vi "TEST Set Wind Speeds - Solution.vi"() -> ()   [LabVIEW 2011]
doc: "Two VI solution that allows the user to test the Wind Turbine class. Speed is set in one VI and read in another.\n\nAAL 9/09"
uses:
  SEQ - Solution.lvlib
panel:
  in  "Exit":bool
  in  "Set Speed":bool
  in  "Turbine":u16(ring) items=["Wind Turbine #1", "Wind Turbine #2", "Wind Turbine #3"]
  in  "Wind Speed (m/s)":dbl
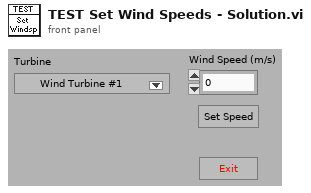
[diagram p1: front panel]
types:
  T1 = typedef "SEQ - Solution.lvlib/Wind Turbine DataRef.ctl" = refnum<queue>
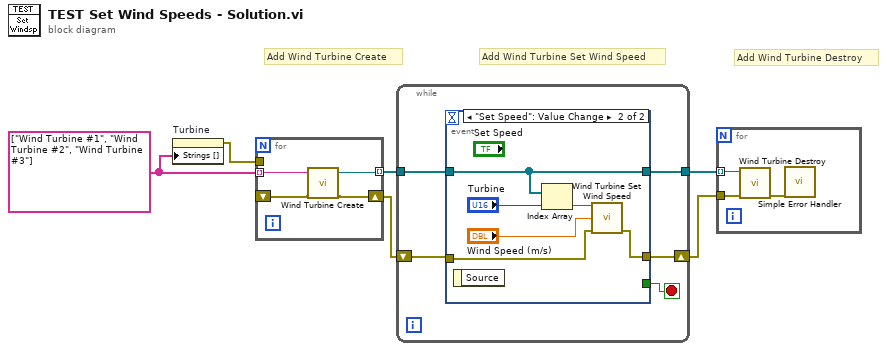
[diagram p0: block diagram]
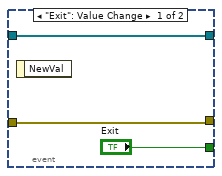
[diagram p2: hidden frame]
diagram:
  w6 = string[] ["Wind Turbine #1", "Wind Turbine #2", "Wind Turbine #3"]
  # "Add Wind Turbine Destroy"
  # "Add Wind Turbine Set Wind Speed"
  # "Add Wind Turbine Create"
  n1 = property on="Turbine" class="Ring (strict)"("Strings []"=w6) -> (error out=w3:errorcluster)  [unwired: 2 in, 1 out]
  n2 = for {
    tunnel: w6 -> [w7] mode=indexing
    tunnel: [w9] -> w5 mode=indexing
    tunnel: w3 -> [_]
    shift-right: [w8] -> w2
    shift-left: _ -> [w10]
    n3 = call "Wind Turbine Create.vi"("error in (no error)"=w10, "SEQ Name"=w7) -> ("error out"=w8:errorcluster, "Data Refnum out"=w9:T1)  [unwired: 8 in]
  }
  n4 = while {
    tunnel: w5 -> [w14]
    tunnel: [w13] -> w4
    shift-right: [w12] -> w1
    shift-left: w2 -> [w11]
    stop <- w15 stop-if-true
    n5 = event shown="[1] \"Set Speed\": Value Change" {
      selector: _ -> [_ _]
      dyn-events: _ -> [_ _]
      timeout: _ -> [_ _]
      tunnel: ["Exit" _] -> w15
      tunnel: w14 -> [w17 w23]
      tunnel: [w17 w23] -> w13
      tunnel: w11 -> [w16 w20]
      tunnel: [w16 w19] -> w12
      event "Exit": Value Change {
        n6 = event-data() -> ()  [unwired: 2 out]
      }
      event "Set Speed": Value Change {
        n7 = event-data() -> ()  [unwired: 2 out]
        n8 = Index Array(array=w23, index="Turbine") -> (element=w22:T1)
        n9 = call "Wind Turbine Set Wind Speed.vi"("Data Refnum"=w22, "Wind Speed (ms)"="Wind Speed (m/s)", "error in (no error)"=w20) -> ("error out"=w19:errorcluster)  [unwired: 11 in, 1 out]
      }
    }
  }
  n10 = for {
    tunnel: w4 -> [w27] mode=indexing
    tunnel: w1 -> [w26]
    n11 = call "Wind Turbine Destroy.vi"("error in (no error)"=w26, "Data Refnum"=w27) -> ("error out"=w25:errorcluster)  [unwired: 8 in, 1 out]
    n12 = call <vilib>:"Simple Error Handler.vi"("error in (no error)"=w25) -> ()  [unwired: 1 in, 8 out]
  }
